vi "Post-Install Custom Action.vi"(10 "Variant":variant) -> (0 "error out":errorcluster)   [LabVIEW 2015]
doc: "<b> </b> <b> </b>\n©2016 Q Software Innovations, LLC (QSI)\nwritten by Quentin Alldredge\nproduced in LabVIEW 2015\n\nsupport@qsoftwareinnovations.com\nwww.qsoftwareinnovations.com\n\nAll rights reserved.\n\nRedistribution and use in source and binary forms, with or without modification, are permitted provided that the following conditions are met:\n\n * Redistributions of source code must retain the above copyright notice, this list of conditions and the following disclaimer.\n * Redistributions in binary form must reproduce the above copyright notice, this list of conditions and the following disclaimer in the documentation and/or other materials provided with the distribution.\n * Neither the name of Q Software Innovations, LLC. nor the names of its contributors may be used to endorse or promote products derived from this software without specific prior written permission.\n\nTHIS SOFTWARE IS PROVIDED BY THE COPYRIGHT HOLDERS AND CONTRIBUTORS \"AS IS\" AND ANY EXPRESS OR IMPLIED WARRANTIES, INCLUDING, BUT NOT LIMITED TO, THE IMPLIED WARRANTIES OF MERCHANTABILITY AND FITNESS FOR A PARTICULAR PURPOSE ARE DISCLAIMED. IN NO EVENT SHALL THE COPYRIGHT OWNER OR CONTRIBUTORS BE LIABLE FOR ANY DIRECT, INDIRECT, INCIDENTAL, SPECIAL, EXEMPLARY, OR CONSEQUENTIAL DAMAGES (INCLUDING, BUT NOT LIMITED TO, PROCUREMENT OF SUBSTITUTE GOODS OR SERVICES; LOSS OF USE, DATA, OR PROFITS; OR BUSINESS INTERRUPTION) HOWEVER CAUSED AND ON ANY THEORY OF LIABILITY, WHETHER IN CONTRACT, STRICT LIABILITY, OR TORT (INCLUDING NEGLIGENCE OR OTHERWISE) ARISING IN ANY WAY OUT OF THE USE OF THIS SOFTWARE, EVEN IF ADVISED OF THE POSSIBILITY OF SUCH DAMAGE."
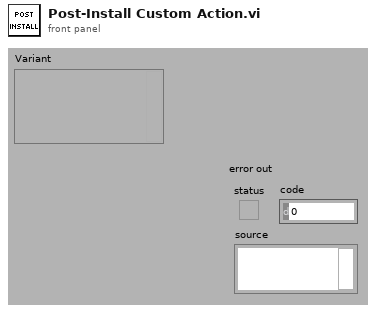
[diagram p1: front panel]
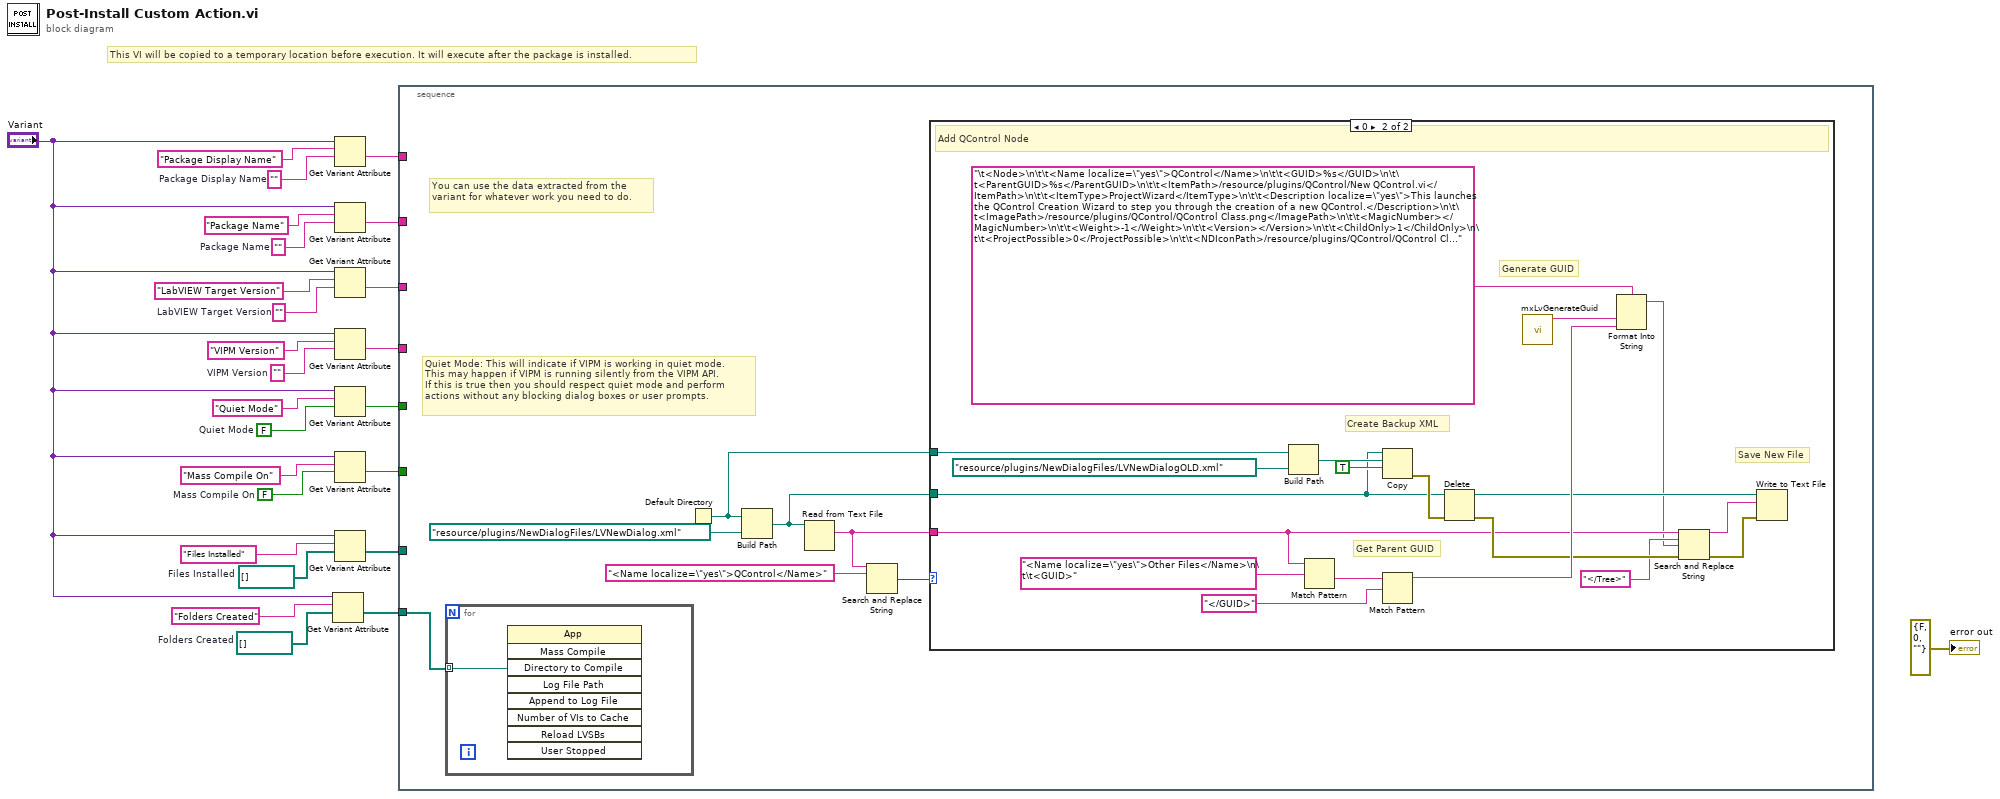
[diagram p0: block diagram]
diagram:
  w1 = path[] []  # Folders Created
  w2 = path[] []  # Files Installed
  w8 = FALSE  # Mass Compile On
  w9 = ""  # Package Display Name
  w16 = FALSE  # Quiet Mode
  w19 = ""  # VIPM Version
  w21 = ""  # LabVIEW Target Version
  w23 = ""  # Package Name
  # "This VI will be copied to a temporary location before execution. It will execute after the package is installed."
  n1 = Get Variant Attribute(Variant="Variant", name="Folders Created", default value (empty Variant)=w1) -> (value=w6:path[])  [unwired: 1 in, 3 out]
  n2 = Get Variant Attribute(Variant="Variant", name="Package Display Name", default value (empty Variant)=w9) -> (value=w15:string)  [unwired: 1 in, 3 out]
  n3 = Get Variant Attribute(Variant="Variant", name="Package Name", default value (empty Variant)=w23) -> (value=w14:string)  [unwired: 1 in, 3 out]
  n4 = Get Variant Attribute(Variant="Variant", name="LabVIEW Target Version", default value (empty Variant)=w21) -> (value=w13:string)  [unwired: 1 in, 3 out]
  n5 = Get Variant Attribute(Variant="Variant", name="VIPM Version", default value (empty Variant)=w19) -> (value=w12:string)  [unwired: 1 in, 3 out]
  n6 = Get Variant Attribute(Variant="Variant", name="Quiet Mode", default value (empty Variant)=w16) -> (value=w11:bool)  [unwired: 1 in, 3 out]
  n7 = Get Variant Attribute(Variant="Variant", name="Mass Compile On", default value (empty Variant)=w8) -> (value=w10:bool)  [unwired: 1 in, 3 out]
  n8 = Get Variant Attribute(Variant="Variant", name="Files Installed", default value (empty Variant)=w2) -> (value=w5:path[])  [unwired: 1 in, 3 out]
  n9 = stacked-sequence {
    tunnel: w15 -> [_]
    tunnel: w14 -> [_]
    tunnel: w13 -> [_]
    tunnel: w12 -> [_]
    tunnel: w11 -> [_]
    tunnel: w10 -> [_]
    tunnel: w5 -> [_]
    tunnel: w6 -> [w27]
    frame #0 {
      # "You can use the data extracted from the variant for whatever work you need to do."
      # "Quiet Mode: This will indicate if VIPM is working in quiet mode.\nThis may happen if VIPM is running silently from the VIPM API.\nIf this is true then you should respect quiet mode and perform\nactions without any blocking dialog boxes or user prompts."
      n10 = for {
        tunnel: w27 -> [w34] mode=indexing
        n11 = invoke class="App" method="Mass Compile"("Directory to Compile"=w34) -> ()  [unwired: 8 in, 9 out]
      }
      n12 = Default Directory() -> (w33:path)
      n13 = Build Path(base path=w33, name or relative path=path "resource/plugins/NewDialogFiles/LVNewDialog.xml") -> (appended path=w29:path)
      n14 = Read from Text File(file (use dialog)=w29) -> (text=w31:string)  [unwired: 3 in, 3 out]
      n15 = Search and Replace String(input string=w31, search string="<Name localize=\"yes\">QControl</Name>") -> (number of replacements=w28:i32)  [unwired: 6 in, 3 out]
      n16 = case shown="0" w28 {
        tunnel: w33 -> [_ w50]
        tunnel: w31 -> [_ w42]
        tunnel: w29 -> [_ w35]
        frame Default {
          # "QControl Node Exists"
        }
        frame 0 {
          # "Save New File"
          # "Generate GUID"
          # "Get Parent GUID"
          # "Create Backup XML"
          # "Add QControl Node"
          n17 = Build Path(base path=w50, name or relative path=path "resource/plugins/NewDialogFiles/LVNewDialogOLD.xml") -> (appended path=w52:path)
          n18 = Match Pattern(string=w42, regular expression="<Name localize=\"yes\">Other Files</Name>\n\t\t<GUID>") -> (after substring=w48:string)  [unwired: 1 in, 3 out]
          n19 = Copy(9:TRUE ("overwrite (F)"), 10:w52, 11:w35) -> (0:w36:errorcluster)  [unwired: 2 in, 2 out]
          n20 = Match Pattern(string=w48, regular expression="</GUID>") -> (before substring=w45:string)  [unwired: 1 in, 3 out]
          n21 = Delete(path (use dialog)=w35, error in=w36) -> (deleted path=w44:path, error out=w43:errorcluster)  [unwired: 3 in, 1 out]
          n22 = call <resource>:"mxLvGenerateGuid.vi"() -> ("Value"=w41:string)  [unwired: 10 in, 1 out]
          n23 = Format Into String(format string="\t<Node>\n\t\t<Name localize=\"yes\">QControl</Name>\n\t\t<GUID>%s</GUID>\n\t\t<ParentGUID>%s</ParentGUID>\n\t\t<ItemPath>/resource/plugins/QControl/New QControl.vi</ItemPath>\n\t\t<ItemType>ProjectWizard</ItemType>\n\t\t<Description localize=\"yes\">This launches the QControl Creation Wizard to step you through the creation of a new QControl.</Description>\n\t\t<ImagePath>/resource/plugins/QControl/QControl Class.png</ImagePath>\n\t\t<MagicNumber></MagicNumber>\n\t\t<Weight>-1</Weight>\n\t\t<Version></Version>\n\t\t<ChildOnly>1</ChildOnly>\n\t\t<ProjectPossible>0</ProjectPossible>\n\t\t<NDIconPath>/resource/plugins/QControl/QControl Class Icon.png</NDIconPath>\n\t</Node>\t \n</Tree>", w41, w45) -> (resulting string=w39:string)  [unwired: 2 in, 1 out]
          n24 = Search and Replace String(input string=w42, search string="</Tree>", replace string=w39, error in=w43) -> (result string=w37:string, error out=w38:errorcluster)  [unwired: 4 in, 2 out]
          n25 = Write to Text File(file (use dialog)=w44, text=w37, error in=w38) -> ()  [unwired: 1 in, 3 out]
        }
      }
    }
  }
  "error out" <- errorcluster {"status"=FALSE, "code"=0, "source"=""} ("error out")
